vi "Zero Padder (DBL).vi"(10 "only non-power of 2?":bool, 11 "Input Array":dbl[](array[numeric])) -> (3 "Zero Padded Array":dbl[](array[numeric]))   [LabVIEW 2017, in "NI_AALPro.lvlib"]
doc: "Resizes the input sequence <B>Input Array</B> to the next higher valid power of 2, sets the new trailing elements of the sequence to zero, and leaves the first n elements unchanged, where n is the number of samples in the input sequence. Wire data to the <B>Input Array</B> input to determine the polymorphic instance to use or manually select the instance."
uses:
  NI_AALPro.lvlib
panel:
  # "Zero Padder (DBL)"
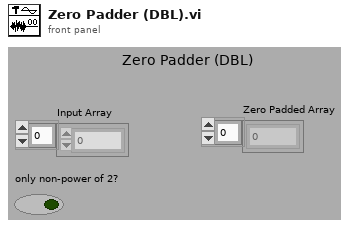
[diagram p1: front panel]
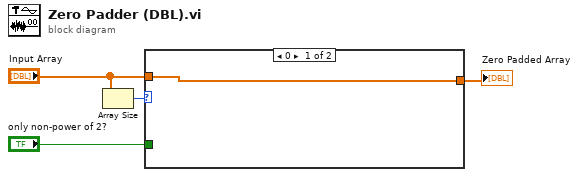
[diagram p0: block diagram]
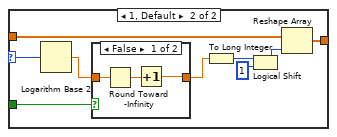
[diagram p2: hidden frame]
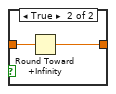
[diagram p3: hidden frame]
diagram:
  n1 = Array Size(array="Input Array") -> (size(s)=w4:i32)
  n2 = case shown="0" w4 {
    selector: w4 -> [_ w9]
    tunnel: "Input Array" -> [w5 w11]
    tunnel: [w5 w10] -> w2
    tunnel: "only non-power of 2?" -> [_ w8]
    frame 0 {
    }
    frame 1, Default {
      n3 = Logarithm Base 2(1:w9) -> (0:w7:dbl)
      n4 = case shown="False" w8 {
        tunnel: w7 -> [w17 w19]
        tunnel: [w15 w18] -> w6
        frame False {
          n5 = Round Toward -Infinity(1:w17) -> (0:w16:dbl)
          n6 = Increment(x=w16) -> (x+1=w15:dbl)
        }
        frame True {
          n7 = Round Toward +Infinity(x=w19) -> (ceil(x): smallest int >= x=w18:dbl)
        }
      }
      n8 = To Long Integer(number=w6) -> (32bit integer=w12:i32)
      n9 = Logical Shift(y=w12, x=1) -> (x << y=w13:i32)
      n10 = Reshape Array(w11, w13) -> (w10:dbl[])
    }
  }
  "Zero Padded Array" <- w2
